vi "Highlight Item.vi"(0 "Display State In":T1={"logTable"=refnum, "max items"=500, "displaydata"=[], "data"=[], "Auto Scroll"=TRUE, "current item"=500, "col headers"=[], "Add to Top"=TRUE, "Auto resize"=TRUE, "col size"=[], "filters"=[], "color cells"=[]}, 1 "Column":string, 2 "Value":string, 9 "Container State":T3, 11 "error in (no error)":errorcluster, 12 "Hightlight Column":string, 13 "Color Box":u32(colorbox)) -> (4 "Display State Out":T1={"logTable"=refnum, "max items"=500, "displaydata"=[], "data"=[], "Auto Scroll"=TRUE, "current item"=500, "col headers"=[], "Add to Top"=TRUE, "Auto resize"=TRUE, "col size"=[], "filters"=[], "color cells"=[]}, 15 "error out":errorcluster)   [LabVIEW 2013, in "UI-DisplayTable(dev).xctl"]
uses:
  UI-DisplayTable(dev).xctl
  <vilib>/_xctls/Container State.ctl
  State.ctl
  Support/DEF-Filter.ctl
  <vilib>/Utility/miscctls.llb/LVRowAndColumnTypeDef.ctl
  <vilib>/_xctls/XControlSupport.lvlib
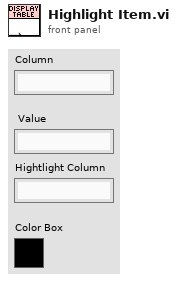
[diagram p1: front panel]
types:
  T1 = typedef "UI-DisplayTable(dev).xctl/State.ctl" = cluster{"logTable":refnum<vi>, "max items":i32, "displaydata":string[][], "data":string[][], "Auto Scroll":bool, "current item":i32, "col headers":string[], "Add to Top":bool, "Auto resize":bool, "col size":i32[], "filters":T2[], "color cells":cluster{"color cell":cluster{"Column":string, "Value":string, "Highlight Column":string}, "Color Box":u32}[]}
  T2 = typedef "UI-DisplayTable(dev).xctl/DEF-Filter.ctl" = cluster{"column":string, "value":string[]}
  T3 = typedef "XControlSupport.lvlib/Container State.ctl" = cluster{"Indicator?":bool, "Run Mode?":bool, " Refnum":refnum<vi>}
  T4 = cluster{"color cell":cluster{"Column":string, "Value":string, "Highlight Column":string}, "Color Box":u32}
  T5 = typedef "LVRowAndColumnTypeDef.ctl" = cluster{"Row":i32, "Column":i32}
  T6 = cluster{"color cell":cluster{"Column":string, "Value":string, "Highlight Column":string}, "Color Box":u32}[]
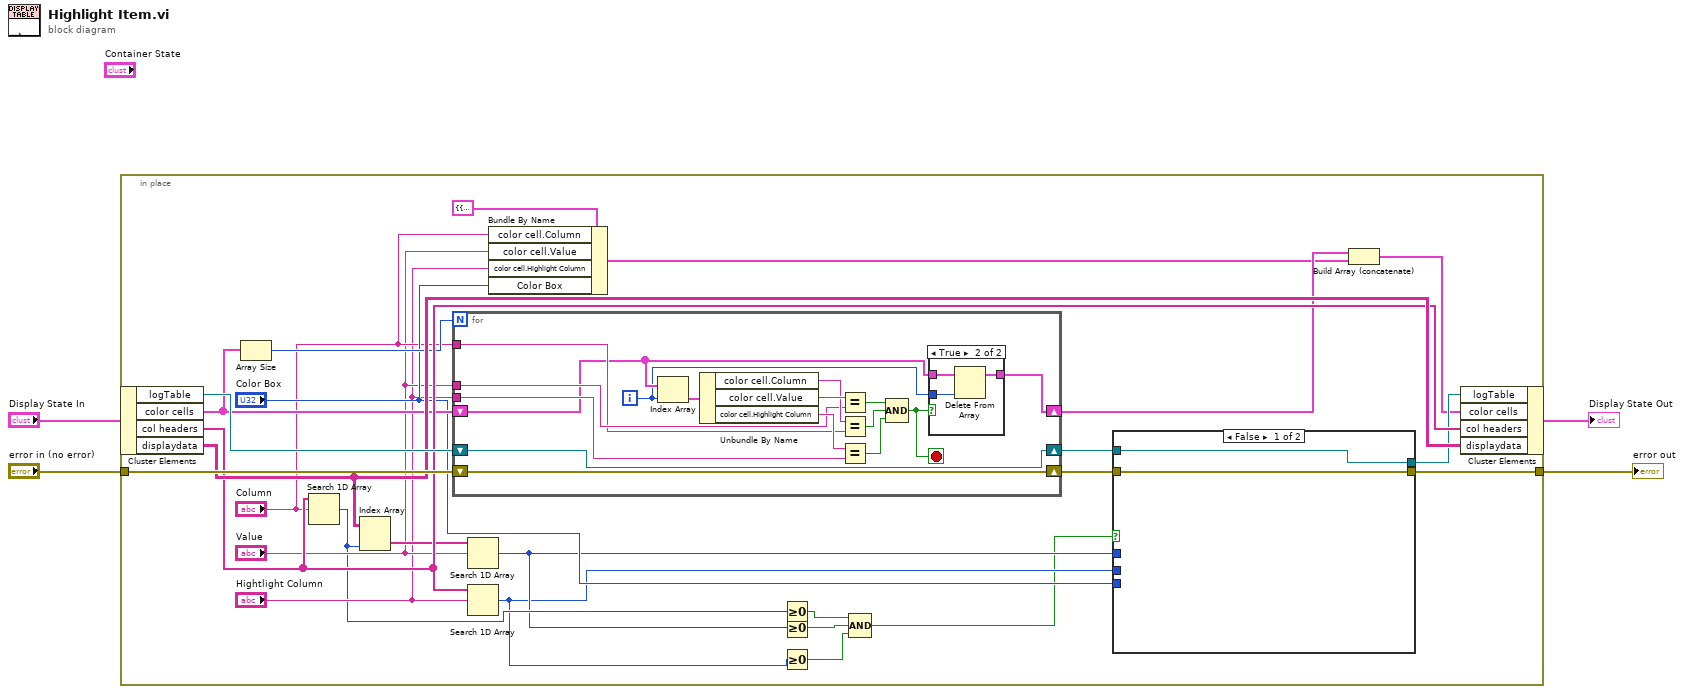
[diagram p0: block diagram]
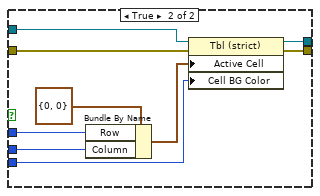
[diagram p2: hidden frame]
diagram:
  n1 = in-place {
    in-place-border: "error in (no error)" -> [w30]
    in-place-border: [w24] -> w3
    n2 = in-place-cluster #1("Display State In") -> ("logTable"=w29:refnum<vi>, "color cells"=w22:T6, "col headers"=w27:string[], "displaydata"=w28:string[][])
    n3 = Array Size(array=w22) -> (size(s)=w21:i32)
    n4 = Search 1D Array(1D array=w27, element="Column") -> (index of element=w8:i32)  [unwired: 1 in]
    n5 = Index Array(array=w28, index (col)=w8) -> (element=w20:string[])  [unwired: 1 in]
    n6 = for {
      N: w21 -> [_]
      shift-right: [w51] -> w25
      shift-left: w30 -> [w51]
      shift-right: [w50] -> w26
      shift-left: w29 -> [w50]
      tunnel: "Value" -> [w49]
      tunnel: "Column" -> [w48]
      tunnel: "Hightlight Column" -> [w47]
      shift-right: [w43] -> w18
      shift-left: w22 -> [w44]
      i -> [w42]
      stop <- w45 stop-if-true
      n7 = Index Array(array=w44, index=w42) -> (element=w46:T4)
      n8 = Unbundle By Name(w46) -> ("color cell.Column"=w54:string, "color cell.Value"=w55:string, "color cell.Highlight Column"=w53:string)
      n9 = Equal?(x=w55, y=w49) -> (x = y?=w56:bool)
      n10 = Equal?(x=w54, y=w48) -> (x = y?=w57:bool)
      n11 = Equal?(x=w53, y=w47) -> (x = y?=w52:bool)
      n12 = Compound Arithmetic op=AND(w56, w57, w52) -> (w45:bool)
      n13 = case shown="True" w45 {
        tunnel: w44 -> [w58 w61]
        tunnel: [w58 w60] -> w43
        tunnel: w42 -> [_ w59]
        frame False {
        }
        frame True {
          n14 = Delete From Array(array=w61, index=w59) -> (array with subset deleted=w60:T6)  [unwired: 1 in, 1 out]
        }
      }
    }
    n15 = Search 1D Array(1D array=w20, element="Value") -> (index of element=w7:i32)  [unwired: 1 in]
    n16 = Search 1D Array(1D array=w27, element="Hightlight Column") -> (index of element=w6:i32)  [unwired: 1 in]
    n17 = Bundle By Name(cluster=T4 {"color cell"={"Column"="", "Value"="", "Highlight Column"=""}, "Color Box"=0} ("element"), "color cell.Column"="Column", "color cell.Value"="Value", "color cell.Highlight Column"="Hightlight Column", "Color Box"="Color Box") -> (w16:T4)
    n18 = Greater Or Equal To 0?(x=w8) -> (x >= 0?=w11:bool)
    n19 = Greater Or Equal To 0?(x=w7) -> (x >= 0?=w10:bool)
    n20 = Greater Or Equal To 0?(x=w6) -> (x >= 0?=w9:bool)
    n21 = Compound Arithmetic op=AND(w11, w10, w9) -> (w5:bool)
    n22 = case shown="False" w5 {
      tunnel: w26 -> [w32 w41]
      tunnel: w25 -> [w31 w40]
      tunnel: [w31 w39] -> w24
      tunnel: [w32 w38] -> w23
      tunnel: "Color Box" -> [_ w35]
      tunnel: w7 -> [_ w34]
      tunnel: w6 -> [_ w33]
      frame False {
      }
      frame True {
        n23 = Bundle By Name(cluster=T5 {"Row"=0, "Column"=0} ("Active Cell:Active Cell"), "Row"=w34, "Column"=w33) -> (w36:T5)
        n24 = property class="Tbl (strict)"(reference=w41, error in=w40, "Active Cell"=w36, "Cell BG Color"=w35) -> (reference out=w38:refnum<vi>, error out=w39:errorcluster)
      }
    }
    n25 = Build Array (concatenate)(w18, w16) -> (w17:T6)
    n26 = in-place-cluster #1("logTable"=w23, "color cells"=w17, "col headers"=w27, "displaydata"=w28) -> (→"Display State Out":T1)
  }
  "error out" <- w3
